vi "Load Animated GIF Image (UTF-8 Path).vi"(8 "error in (no error)":errorcluster, 11 "Path In":string) -> (0 "error out":errorcluster, 1 "Delays":i32[](array[numeric]), 2 "Frames":T1[](array[typedef]), 3 "Path Out":string)   [LabVIEW 2020, in "G-Image.lvlib"]
doc: "Load an animated GIF image file from disk and return it as an array of LabVIEW pictures.\n\nThe Delays array are the times in milliseconds to display each frame, and can vary between frames.\n\nNote this function can load non-animated GIF types, which are returned as a single frame."
uses:
  G-Image.lvlib
  <vilib>/picture/picture.llb/imagedata.ctl
  Private/Result To Error.vi
  <vilib>/Utility/error.llb/Error Cluster From Error Code.vi
  Private/Copy Image To Picture.vi
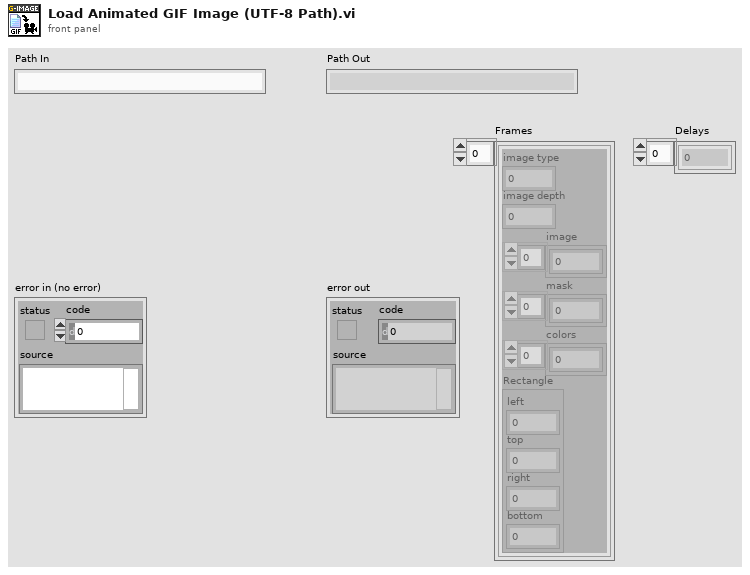
[diagram p1: front panel]
types:
  T1 = typedef "imagedata.ctl" = cluster{"image type":i32, "image depth":i32, "image":u8[], "mask":u8[], "colors":u32[], "Rectangle":cluster{"left":i16, "top":i16, "right":i16, "bottom":i16}}
  T2 = typedef "G-Image.lvlib/Extended Image.ctl" = cluster{"Image":T1, "Layers":i32, "Delays":i32[]}
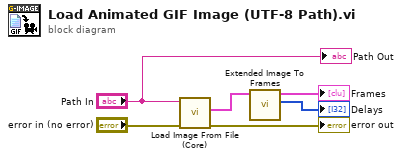
[diagram p0: block diagram]
diagram:
  n1 = call "Load Image From File (Core).vi"("error in (no error)"="error in (no error)", "Path In"="Path In") -> ("error out"=→"error out":errorcluster, "Extended Image"=w1:T2)  [unwired: 7 in, 1 out]
  n2 = call "Extended Image To Frames.vi"("Extended Image"=w1) -> ("Delays"=→"Delays":i32[], "Frames"=→"Frames":T1[])  [unwired: 9 in]
  "Path Out" <- "Path In"
